vi "Pico close.vi"(10 "?":bool, 11 "handle":i16) -> ()   [LabVIEW 2015]
uses:
  Program Files (x86)/Pico Technology/SDK/lib/usbtc08.dll
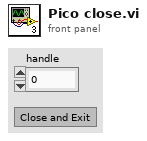
[diagram p1: front panel]
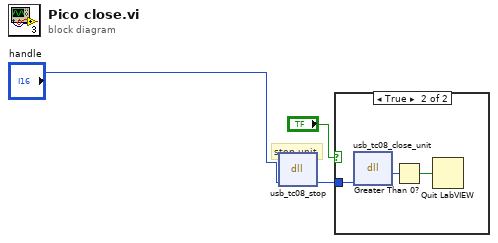
[diagram p0: block diagram]
diagram:
  # "stop unit"
  n1 = dll-call lib="C:/Program Files (x86)/Pico Technology/SDK/lib/usbtc08.dll" fn="usb_tc08_stop" ("Close unit")("handle"="handle") -> ("handle"=w1:i16)  [unwired: 4 in, 2 out]
  n2 = case shown="True" "?" {
    tunnel: w1 -> [_ w6]
    frame False {
    }
    frame True {
      n3 = dll-call lib="C:/Program Files (x86)/Pico Technology/SDK/lib/usbtc08.dll" fn="usb_tc08_close_unit" ("Close unit")("handle"=w6) -> ("return type"=w5:i16)  [unwired: 4 in, 2 out]
      n4 = Greater Than 0?(x=w5) -> (x > 0?=w4:bool)
      n5 = Quit LabVIEW(quit? (T)=w4) -> ()
    }
  }
